vi "xwpfDocument Tests Duplicate Content.vi"() -> ()   [LabVIEW 2017]
uses:
  src/LabVIEW NPOI/xwpfDocument/xwpfDocument.lvclass/xwpfDocument.ctl
  src/LabVIEW NPOI/xwpfDocument/Get Elements.vi
  src/LabVIEW NPOI/xwpfDocument/Get Elements.Text.vi
  src/LabVIEW NPOI/xwpfDocument.Element/xwpfDocument.Element.lvclass
  src/LabVIEW NPOI/xwpfDocument/xwpfDocument.lvclass
panel:
  out "Document:Elements:Text":string[](array[string])
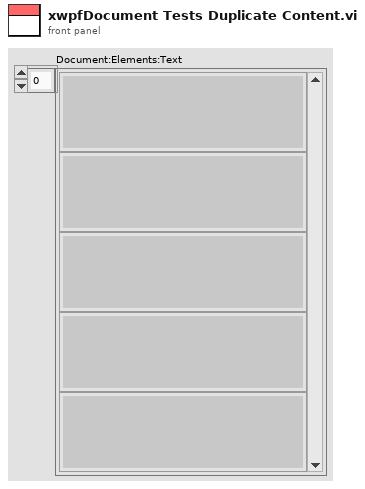
[diagram p1: front panel]
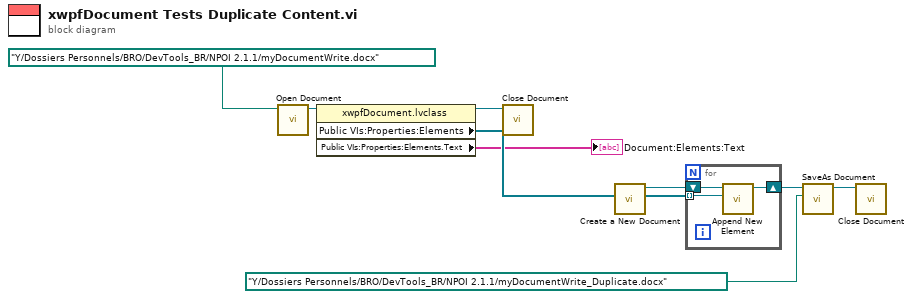
[diagram p0: block diagram]
diagram:
  n1 = call "Open Document.vi"("Document Path"=path "Y:/Dossiers Personnels/BRO/DevTools_BR/NPOI 2.1.1/myDocumentWrite.docx") -> ("xwpfDocument out"=w9:refnum<class "xwpfDocument.lvclass">)  [unwired: 9 in, 1 out]
  n2 = property class="xwpfDocument.lvclass"(reference=w9) -> (reference out=w7:refnum<class "xwpfDocument.lvclass">, "Public VIs:Properties:Elements"=w5:refnum<class "xwpfDocument.Element.lvclass">[], "Public VIs:Properties:Elements.Text"=→"Document:Elements:Text":string[])  [unwired: 1 in, 1 out]
  n3 = call "Close Document.vi"("xwpfDocument in"=w7) -> ()  [unwired: 9 in, 2 out]
  n4 = call "Create a New Document.vi"() -> ("xwpfDocument out"=w6:refnum<class "xwpfDocument.lvclass">)  [unwired: 10 in, 1 out]
  n5 = for {
    shift-right: [w11] -> w4
    shift-left: w6 -> [w12]
    tunnel: w5 -> [w10] mode=indexing
    n6 = call "Append New Element.vi"("New Element"=w10, "xwpfDocument in"=w12) -> ("xwpfDocument out"=w11:refnum<class "xwpfDocument.lvclass">)  [unwired: 8 in, 1 out]
  }
  n7 = call "SaveAs Document.vi"("Document Path"=path "Y:/Dossiers Personnels/BRO/DevTools_BR/NPOI 2.1.1/myDocumentWrite_Duplicate.docx", "xwpfDocument in"=w4) -> ("xwpfDocument out"=w3:refnum<class "xwpfDocument.lvclass">)  [unwired: 8 in, 1 out]
  n8 = call "Close Document.vi"("xwpfDocument in"=w3) -> ()  [unwired: 9 in, 2 out]
